vi "Oqus Initialization VI.vi"(8 "error in (no error)":errorcluster, 10 "Custom XML":string, 11 "Device Item Ref in":T1 format="%.0x") -> (0 "error out":errorcluster, 3 "Device Item Ref out":T1 format="%.0x")   [LabVIEW 2013, in "Oqus Custom Device.lvlib"]
uses:
  Oqus Custom Device.lvlib
  <vilib>/NI Veristand/Custom Device API/Custom Device Item Ref.ctl
  <vilib>/NI Veristand/Custom Device API/Custom Device Channel.ctl
  <vilib>/NI Veristand/Custom Device API/Custom Device Channel Type.ctl
  <vilib>/NI Veristand/Custom Device API/Custom Device API.lvlib
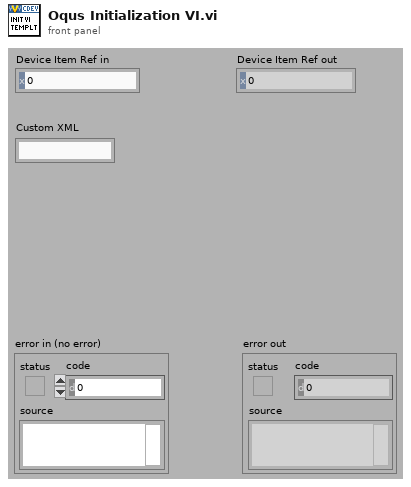
[diagram p1: front panel]
types:
  T1 = typedef "Custom Device API.lvlib/Custom Device Item Ref.ctl" = u64
  T2 = typedef "Custom Device API.lvlib/Custom Device Channel.ctl" = cluster{"Type":T3, "Units":string, "Default Value":dbl, "Faultable":bool, "Scalable":bool}
  T3 = typedef "Custom Device API.lvlib/Custom Device Channel Type.ctl" = enum16{"Input", "Output"}
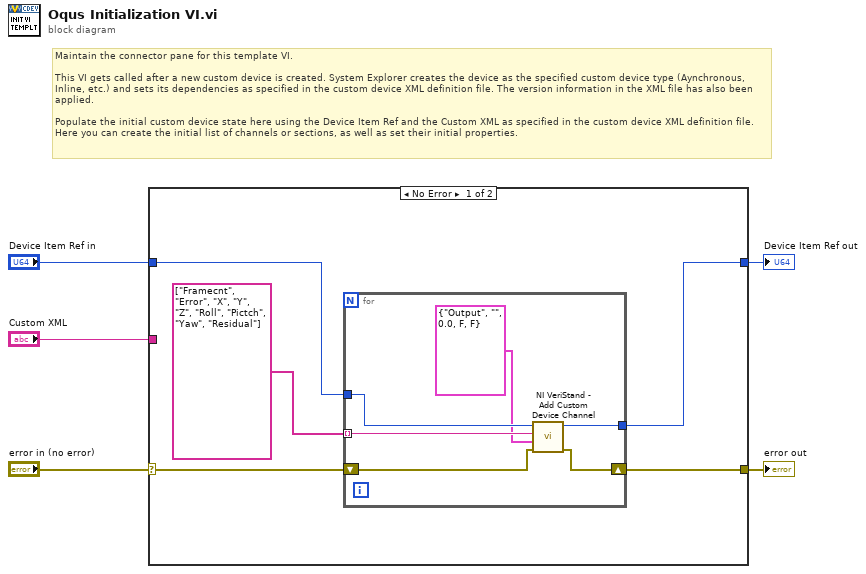
[diagram p0: block diagram]
diagram:
  # "Maintain the connector pane for this template VI.\n\nThis VI gets called after a new custom device is created. System Explorer creates the device as the specified custom device type (Aynchronous, Inline, etc.) and sets its dependencies as specified in the custom device XML definition file. The version information in the XML file has also been applied.\n\nPopulate the initial custom device state here using the Device Item Ref and the Custom XML as specified in the custom device XML definition file. Here you can create the initial list of channels or sections, as well as set their initial properties."
  n1 = case shown="No Error" "error in (no error)" {
    selector: "error in (no error)" -> [w8 w18]
    tunnel: [w7 w18] -> w5
    tunnel: [w6 w17] -> w3
    tunnel: "Device Item Ref in" -> [w10 w17]
    tunnel: "Custom XML" -> [_ _]
    frame No Error {
      n2 = for {
        tunnel: w10 -> [w16]
        tunnel: string[] ["Framecnt", "Error", "X", "Y", "Z", "Roll", "Pictch", "Yaw", "Residual"] -> [w15] mode=indexing
        shift-right: [w12] -> w7
        shift-left: w8 -> [w13]
        tunnel: [w11] -> w6
        n3 = call <vilib>:"NI VeriStand - Add Custom Device Channel.vi"("error in (no error)"=w13, "Channel"=T2 {"Type"=enum."Output", "Units"="", "Default Value"=0.0, "Faultable"=FALSE, "Scalable"=FALSE}, "Channel Name"=w15, "Parent Ref in"=w16) -> ("error out"=w12:errorcluster, "Parent Ref out"=w11:T1)  [unwired: 4 in, 2 out]
      }
    }
    frame Error {
    }
  }
  "error out" <- w5
  "Device Item Ref out" <- w3
